vi "Shift Redgeister Set to Zero SubVI.vi"() -> ()   [LabVIEW 2020]
uses:
  <vilib>/DAQmx/write.llb/DAQmx Write (Digital Bool 1Line 1Point).vi
  <vilib>/DAQmx/create/channels.llb/DAQmx Create Channel (DO-Digital Output).vi
  <vilib>/DAQmx/miscellaneous.llb/DAQmx Fill In Error Info.vi
panel:
  in  "Clear Pin Task In 2":refnum<k21>
  out "Clear Pin Task Out 2":refnum<k21>
  out "Sync Pin Task Out":refnum<k21>
  in  "Sync Pin Task In":refnum<k21>
  out "Clear Pin Task Out":refnum<k21>
  in  "Clear Pin Task In":refnum<k21>
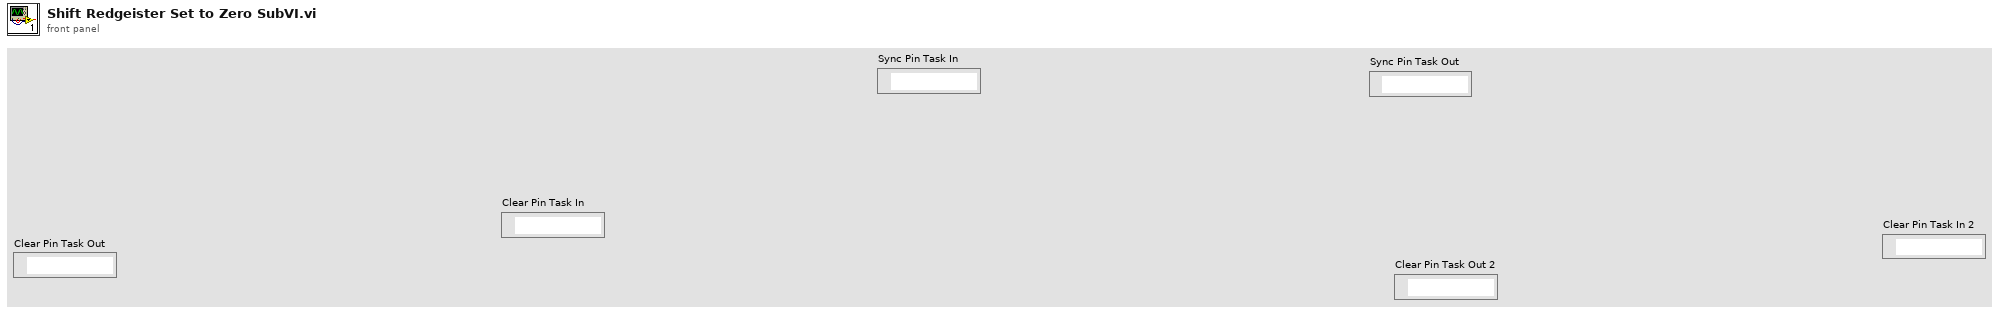
[diagram p1: front panel]
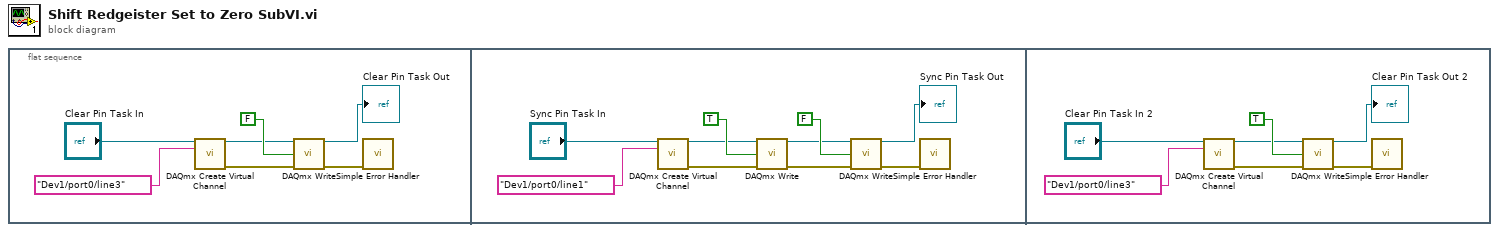
[diagram p0: block diagram]
diagram:
  n1 = flat-sequence {
    frame #0 {
      n2 = call-poly <vilib>:"DAQmx Create Virtual Channel.vi"("task in"="Clear Pin Task In", "lines"=tag "Dev1/port0/line3") -> ("task out"=w3:refnum<k21>, "error out"=w2:errorcluster)  [unwired: 12 in]
      n3 = call-poly <vilib>:"DAQmx Write.vi"("task/channels in"=w3, "data"=FALSE, "error in"=w2) -> ("task out"=→"Clear Pin Task Out":refnum<k21>, "error out"=w5:errorcluster)  [unwired: 10 in, 1 out]
      n4 = call <vilib>:"Simple Error Handler.vi"("error in (no error)"=w5) -> ()  [unwired: 4 in, 5 out]
    }
    frame #1 {
      n5 = call-poly <vilib>:"DAQmx Create Virtual Channel.vi"("task in"="Sync Pin Task In", "lines"=tag "Dev1/port0/line1") -> ("task out"=w10:refnum<k21>, "error out"=w9:errorcluster)  [unwired: 12 in]
      n6 = call-poly <vilib>:"DAQmx Write.vi"("task/channels in"=w10, "data"=TRUE, "error in"=w9) -> ("task out"=w12:refnum<k21>, "error out"=w13:errorcluster)  [unwired: 10 in, 1 out]
      n7 = call-poly <vilib>:"DAQmx Write.vi"("task/channels in"=w12, "data"=FALSE, "error in"=w13) -> ("task out"=→"Sync Pin Task Out":refnum<k21>, "error out"=w14:errorcluster)  [unwired: 10 in, 1 out]
      n8 = call <vilib>:"Simple Error Handler.vi"("error in (no error)"=w14) -> ()  [unwired: 4 in, 5 out]
    }
    frame #2 {
      n9 = call-poly <vilib>:"DAQmx Create Virtual Channel.vi"("task in"="Clear Pin Task In 2", "lines"=tag "Dev1/port0/line3") -> ("task out"=w20:refnum<k21>, "error out"=w19:errorcluster)  [unwired: 12 in]
      n10 = call-poly <vilib>:"DAQmx Write.vi"("task/channels in"=w20, "data"=TRUE, "error in"=w19) -> ("task out"=→"Clear Pin Task Out 2":refnum<k21>, "error out"=w22:errorcluster)  [unwired: 10 in, 1 out]
      n11 = call <vilib>:"Simple Error Handler.vi"("error in (no error)"=w22) -> ()  [unwired: 4 in, 5 out]
    }
  }
